vi "Do.vi"(8 "error in (no error)":errorcluster, 10 "Actor in":refnum<class "Actor.lvclass">, 11 "Message Template":refnum<class "Initialize Reference Lasers Msg.lvclass">) -> (0 "error out":errorcluster, 2 "Actor out":refnum<class "Actor.lvclass">)   [LabVIEW 2018, in "Range Controller.lvlib" / "Initialize Reference Lasers Msg.lvclass"]
doc: "(<B>Filename</B>: Actor Framework.lvlib:Message.lvclass:Do.vi)\n\nDefines what a message does when it is received by an actor. Generally, a message instructs an actor to invoke one of its methods. By default, this method does nothing. A child class must override it to define behavior. Create a child class by using the Actor Framework Message Maker dialog box."
uses:
  Initialize Reference Lasers Msg.lvclass
  <vilib>/ActorFramework/Actor/Actor.lvclass
  Range Controller Actor.lvclass
  C:/Program Files (x86)/National Instruments/LabVIEW 2018/vi.lib/ActorFramework/Actor/Actor.lvclass
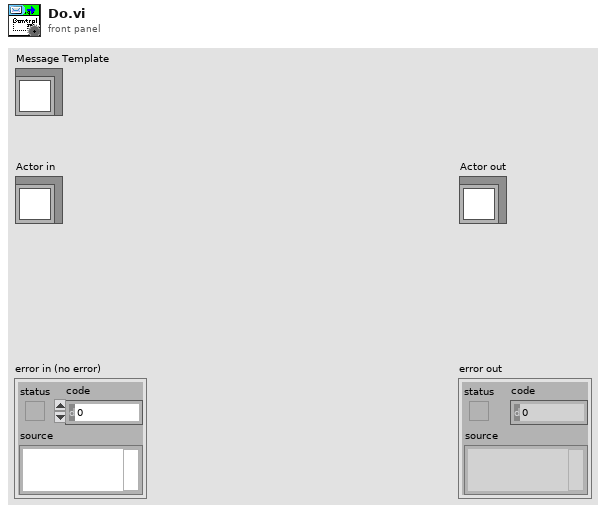
[diagram p1: front panel]
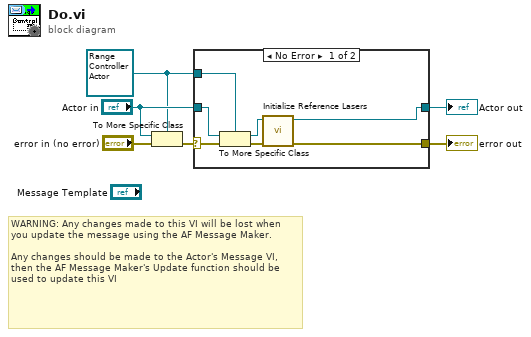
[diagram p0: block diagram]
diagram:
  w1 = refnum<class "Range Controller Actor.lvclass"> refnum ("Actor Type")
  # "WARNING: Any changes made to this VI will be lost when you update the message using the AF Message Maker.\n\nAny changes should be made to the Actor's Message VI, then the AF Message Maker's Update function should be used to update this VI"
  n1 = To More Specific Class(target class=w1, reference="Actor in", error in="error in (no error)") -> (error out=w5:errorcluster)  [unwired: 1 out]
  n2 = case shown="No Error" w5 {
    selector: w5 -> [w13 w15]
    tunnel: [w8 w15] -> w4
    tunnel: [w7 w14] -> w3
    tunnel: "Actor in" -> [w12 w14]
    tunnel: w1 -> [w11 _]
    frame No Error {
      n3 = To More Specific Class ("Actor Cast")(target class=w11, reference=w12, error in=w13) -> (specific class reference=w10:refnum<class "Range Controller Actor.lvclass">, error out=w9:errorcluster)
      n4 = call "Initialize Reference Lasers.vi"("error in (no error)"=w9, "Range Controller Actor in"=w10) -> ("error out"=w8:errorcluster, "Range Controller Actor out"=w7:refnum<class "Range Controller Actor.lvclass">)  [unwired: 8 in]
    }
    frame Error {
    }
  }
  "error out" <- w4
  "Actor out" <- w3
